vi "字符串过滤-正则表达式.vi"(6 "正则式（非汉字单字符）":string="[0-9a-zA-Z_.,]", 11 "字符串 i":string="1234f将6") -> (0 "全匹配？":bool, 3 "字符串 o":string)   [LabVIEW 2017]
doc: "仅用于 单字符（非汉字）的字符串过滤，输入正则表达式是用来判断每一个字节，例如可以是 \"[0-9]\" 不可以用 \"[0-9]+\"。"
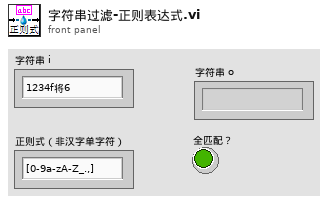
[diagram p1: front panel]
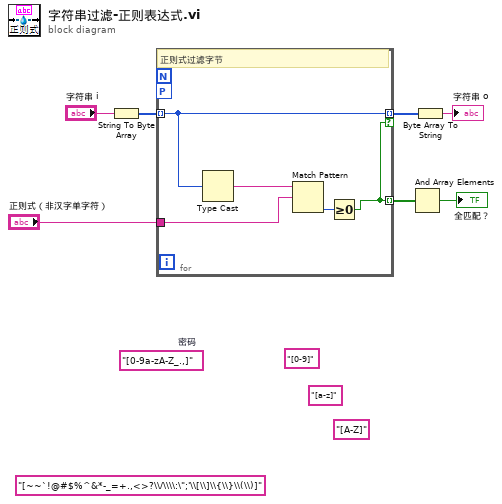
[diagram p0: block diagram]
diagram:
  (unwired) "[~~`!@#$%^&*-_=+.,<>?\\/\\\\:\";'\\[\\]\\{\\}\\(\\)]"
  (unwired) "[0-9a-zA-Z_.,]"  # 密码
  (unwired) "[A-Z]" ("正则表达式")
  (unwired) "[a-z]" ("正则表达式")
  (unwired) "[0-9]" ("正则表达式")
  n1 = String To Byte Array(string="字符串 i") -> (unsigned byte array=w6:u8[])
  n2 = for {
    tunnel: w6 -> [w12] mode=indexing
    tunnel: [w12] -> w5 mode=indexing if=w11
    tunnel: [w11] -> w3 mode=indexing
    tunnel: "正则式（非汉字单字符）" -> [w10]
    workers-P: _ -> [_]
    # "正则式过滤字节"
    n3 = Type Cast(x=w12) -> (*(type *) &x=w9:string)  [unwired: 1 in]
    n4 = Match Pattern(string=w9, regular expression=w10) -> (offset past match=w8:i32)  [unwired: 1 in, 3 out]
    n5 = Greater Or Equal To 0?(x=w8) -> (x >= 0?=w11:bool)
  }
  n6 = And Array Elements(Boolean array=w3) -> (logical AND=→"全匹配？":bool)
  n7 = Byte Array To String(unsigned byte array=w5) -> (string=→"字符串 o":string)
